vi "FileSerialize.vi"(8 "error in (no error)":errorcluster, 10 "DestinationFolder":path, 11 "DocumentType in":refnum<class "Document.lvclass">) -> (0 "error out":errorcluster, 3 "DocumentType out":refnum<class "Document.lvclass">)   [LabVIEW 2021, in "ProligentXMLGenerator.lvlib" / "Document.lvclass"]
uses:
  Document.lvclass
  Document.lvclass/Document.ctl
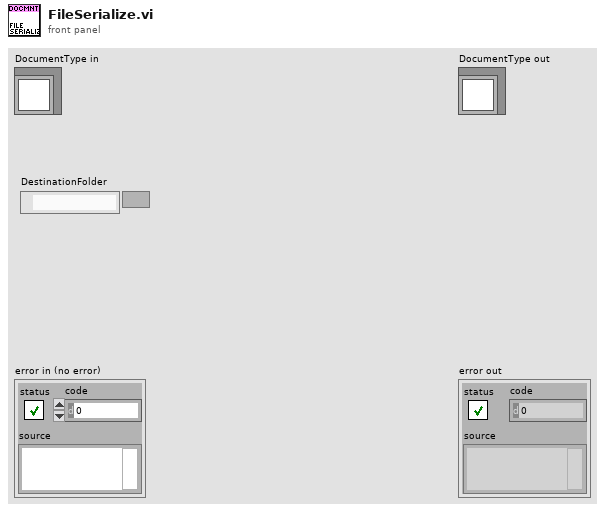
[diagram p1: front panel]
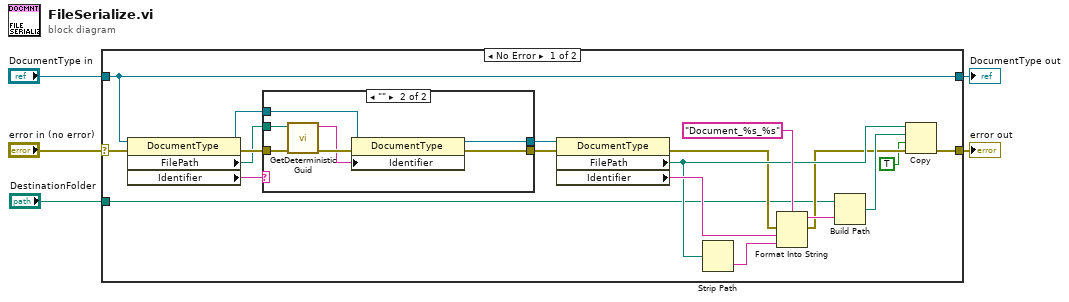
[diagram p0: block diagram]
diagram:
  n1 = case shown="No Error" "error in (no error)" {
    selector: "error in (no error)" -> [w23 w35]
    tunnel: [w15 w35] -> w4
    tunnel: [w24 w34] -> w2
    tunnel: "DocumentType in" -> [w24 w34]
    tunnel: "DestinationFolder" -> [w6 _]
    frame No Error {
      n2 = property on="Property Node" class="DocumentType"(reference=w24, error in=w23) -> (reference out=w20:refnum<class "Document.lvclass">, error out=w22:errorcluster, "FilePath"=w21:path, "Identifier"=w7:string)
      n3 = case shown="\"\"" w7 {
        tunnel: w21 -> [_ w33]
        tunnel: w22 -> [w26 w32]
        tunnel: [w26 w30] -> w18
        tunnel: w20 -> [w25 w29]
        tunnel: [w25 w28] -> w19
        frame Default {
        }
        frame "" {
          n4 = call "GetDeterministicGuid.vi"("error in"=w32, "FilePath"=w33) -> ("error out"=w31:errorcluster, "GUID"=w27:string)  [unwired: 8 in]
          n5 = property on="Property Node" class="DocumentType"(reference=w29, error in=w31, "Identifier"=w27) -> (reference out=w28:refnum<class "Document.lvclass">, error out=w30:errorcluster)
        }
      }
      n6 = property on="Property Node" class="DocumentType"(reference=w19, error in=w18) -> (error out=w10:errorcluster, "FilePath"=w12:path, "Identifier"=w14:string)  [unwired: 1 out]
      n7 = Strip Path(path=w12) -> (name=w11:string)  [unwired: 1 out]
      n8 = Format Into String(format string="Document_%s_%s", error in=w10, w14, w11) -> (resulting string=w17:string, error out=w9:errorcluster)  [unwired: 1 in]
      n9 = Build Path(base path=w6, name or relative path=w17) -> (appended path=w16:path)
      n10 = Copy(8:w9, 9:TRUE ("overwrite (F)"), 10:w16, 11:w12) -> (0:w15:errorcluster)  [unwired: 1 in, 2 out]
    }
    frame Error {
    }
  }
  "error out" <- w4
  "DocumentType out" <- w2
